vi "RelayAction to RelayPosition.vi"(10 "relay action":T2=21 items=["CloseRelay"=21, "OpenRelay"=20]) -> (2 "relay position":T1)   [LabVIEW 2016, in "SLSC Switch.lvlib" / "Relay.lvclass"]
uses:
  Relay.lvclass
  Relay Action.ctl
  Relay Position.ctl
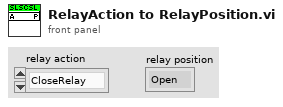
[diagram p1: front panel]
types:
  T1 = typedef "SLSC Switch.lvlib/Relay.lvclass/Relay Position.ctl" = enum16{"Open", "Closed"}
  T2 = typedef "SLSC Switch.lvlib/Relay.lvclass/Relay Action.ctl" = u32
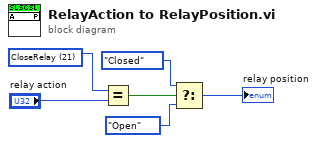
[diagram p0: block diagram]
diagram:
  w5 = T2 21 items=["CloseRelay"=21, "OpenRelay"=20] ("relay action")
  n1 = Equal?(x=w5, y="relay action") -> (x = y?=w6:bool)
  n2 = Select(t=Relay_Position."Closed" ("position"), s=w6, f=Relay_Position."Open" ("position")) -> (s? t:f=→"relay position":T1)
